vi "getCommandID.vi"(8 "error in":errorcluster, 11 "SALCommand.lvclass in":refnum<class "SALCommand.lvclass">) -> (0 "error out":errorcluster, 2 "CommandID":dbl, 3 "SALCommand.lvclass out":refnum<class "SALCommand.lvclass">)   [LabVIEW 2016, in "SALCommand.lvclass"]
uses:
  SALCommand.lvclass
  SALCommand.lvclass/SALCommand.ctl
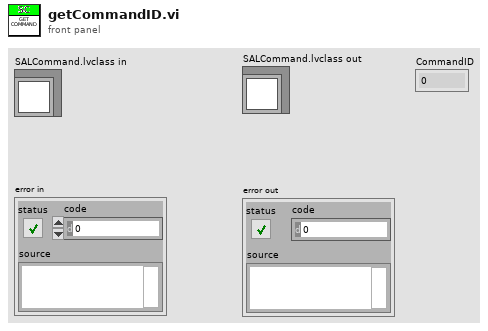
[diagram p1: front panel]
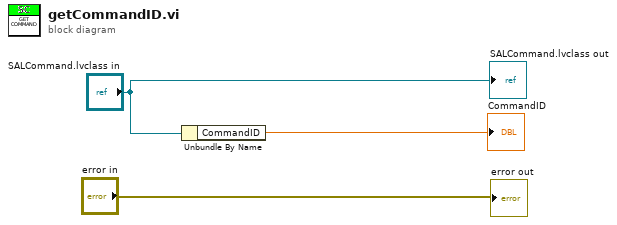
[diagram p0: block diagram]
diagram:
  n1 = Unbundle By Name("SALCommand.lvclass in") -> ("CommandID"=→"CommandID":dbl)
  "SALCommand.lvclass out" <- "SALCommand.lvclass in"
  "error out" <- "error in"
